vi "SizeUp.vi"() -> ()   [LabVIEW 2024, in "TypedCircularBuffer.Tests.Units.lvlib"]
uses:
  TypedCircularBuffer.Tests.Units.lvlib
  <vilib>/addons/_JKI Toolkits/Caraya/classes/Assert/Assert.lvclass
  TypedCircularBuffer.lvclass
  <vilib>/addons/_JKI Toolkits/Caraya/classes/Assert/Assert True.vi
  <vilib>/addons/_JKI Toolkits/Caraya/classes/Assert/Assert Equal Value_Variant.vi
  <vilib>/addons/_JKI Toolkits/Caraya/classes/Assert/Assert Equal Value and Type_Variant.vi
  <vilib>/addons/_JKI Toolkits/Caraya/classes/Assert/Assert False.vi
  <vilib>/addons/_JKI Toolkits/Caraya/classes/Test/Test.lvclass
  Type.ctl
panel:
  in  "Size up Add Expected":T1[](array[typedef])=[0, 1, 2, 3, 4, 5, 6, 7, 8, 9, 255]
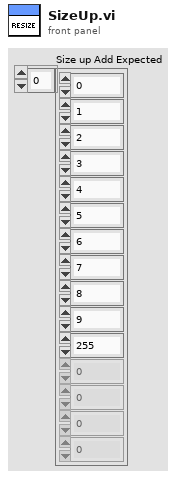
[diagram p1: front panel]
types:
  T1 = typedef "TypedCircularBuffer.lvclass/Type.ctl" = i32
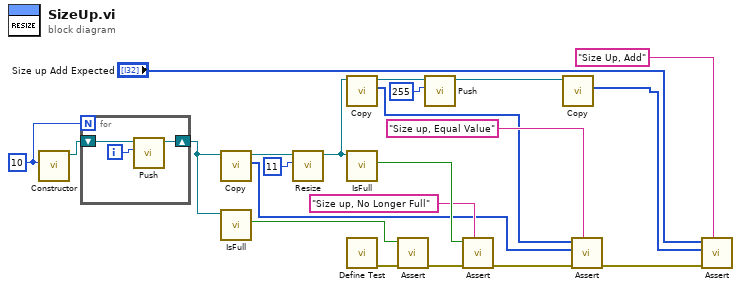
[diagram p0: block diagram]
diagram:
  w7 = u32 10 ("Capacity")
  n1 = call "Constructor.vi"("Capacity"=w7) -> ("TypedCircularBuffer out"=w6:refnum<class "TypedCircularBuffer.lvclass">)  [unwired: 10 in]
  n2 = for {
    N: w7 -> [_]
    shift-right: [w24] -> w5
    shift-left: w6 -> [w25]
    i -> [w23]
    n3 = call "Push.vi"("Element"=w23, "TypedCircularBuffer in"=w25) -> ("TypedCircularBuffer out"=w24:refnum<class "TypedCircularBuffer.lvclass">)  [unwired: 7 in, 2 out]
  }
  n4 = call "Copy.vi"("TypedCircularBuffer in"=w5) -> ("Copied Buffer"=w13:T1[], "TypedCircularBuffer out"=w18:refnum<class "TypedCircularBuffer.lvclass">)  [unwired: 9 in]
  n5 = call "IsFull.vi"("TypedCircularBuffer in"=w5) -> ("Full?"=w21:bool)  [unwired: 9 in, 1 out]
  n6 = call "Resize.vi"("Capacity"=u32 11, "TypedCircularBuffer in"=w18) -> ("TypedCircularBuffer out"=w17:refnum<class "TypedCircularBuffer.lvclass">)  [unwired: 9 in]
  n7 = call "Copy.vi"("TypedCircularBuffer in"=w17) -> ("Copied Buffer"=w1:T1[], "TypedCircularBuffer out"=w12:refnum<class "TypedCircularBuffer.lvclass">)  [unwired: 9 in]
  n8 = call "IsFull.vi"("TypedCircularBuffer in"=w17) -> ("Full?"=w19:bool)  [unwired: 9 in, 1 out]
  n9 = call <vilib>:"Define Test.vi"() -> ("error out"=w4:errorcluster)  [unwired: 10 in, 1 out]
  n10 = call-poly <vilib>:"Assert.vi"("error in (no error)"=w4, "True?"=w21) -> ("error out"=w20:errorcluster)  [unwired: 8 in, 1 out]
  n11 = call "Push.vi"("Element"=u8 255, "TypedCircularBuffer in"=w12) -> ("TypedCircularBuffer out"=w10:refnum<class "TypedCircularBuffer.lvclass">)  [unwired: 7 in, 2 out]
  n12 = call-poly <vilib>:"Assert.vi"("Label"="Size up, No Longer Full", "error in (no error)"=w20, "False?"=w19) -> ("error out"=w16:errorcluster)  [unwired: 7 in, 1 out]
  n13 = call "Copy.vi"("TypedCircularBuffer in"=w10) -> ("Copied Buffer"=w2:T1[])  [unwired: 9 in, 1 out]
  n14 = call-poly <vilib>:"Assert.vi"("Label"="Size up, Equal Value", "error in (no error)"=w16, "Y"=w13, "X"=w1) -> ("error out"=w3:errorcluster)  [unwired: 6 in, 1 out]
  n15 = call-poly <vilib>:"Assert.vi"("Label"="Size Up, Add", "error in (no error)"=w3, "Y"=w2, "X"="Size up Add Expected") -> ()  [unwired: 6 in, 2 out]
